vi "DeviceRead.vi"(4 "等待时间（毫秒）":u32, 5 "VISA resource name":refnum<visa-resource-name> caption="VISA资源名称", 6 "写入缓冲区":string, 7 "标准码词":string) -> (0 "错误输出":errorcluster, 1 "x = y?":bool, 2 "数据读取时间":u32, 3 "连接的字符串":string)   [LabVIEW 2020]
uses:
  <vilib>/Instr/_visa.llb/VISA Flush IO Buffer Mask.ctl
  <vilib>/Instr/_visa.llb/VISA Set IO Buffer Mask.ctl
  <vilib>/Instr/_visa.llb/VISA Configure Serial Port (Instr).vi
panel:
  out "读取的数据":string
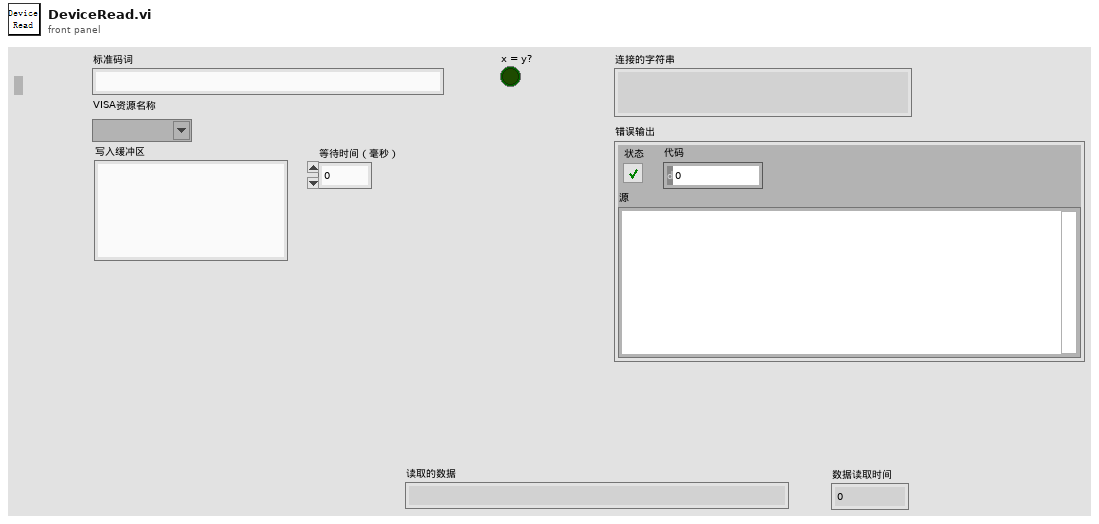
[diagram p1: front panel]
types:
  T1 = typedef "VISA Flush IO Buffer Mask.ctl" = u16
  T2 = typedef "VISA Set IO Buffer Mask.ctl" = u16
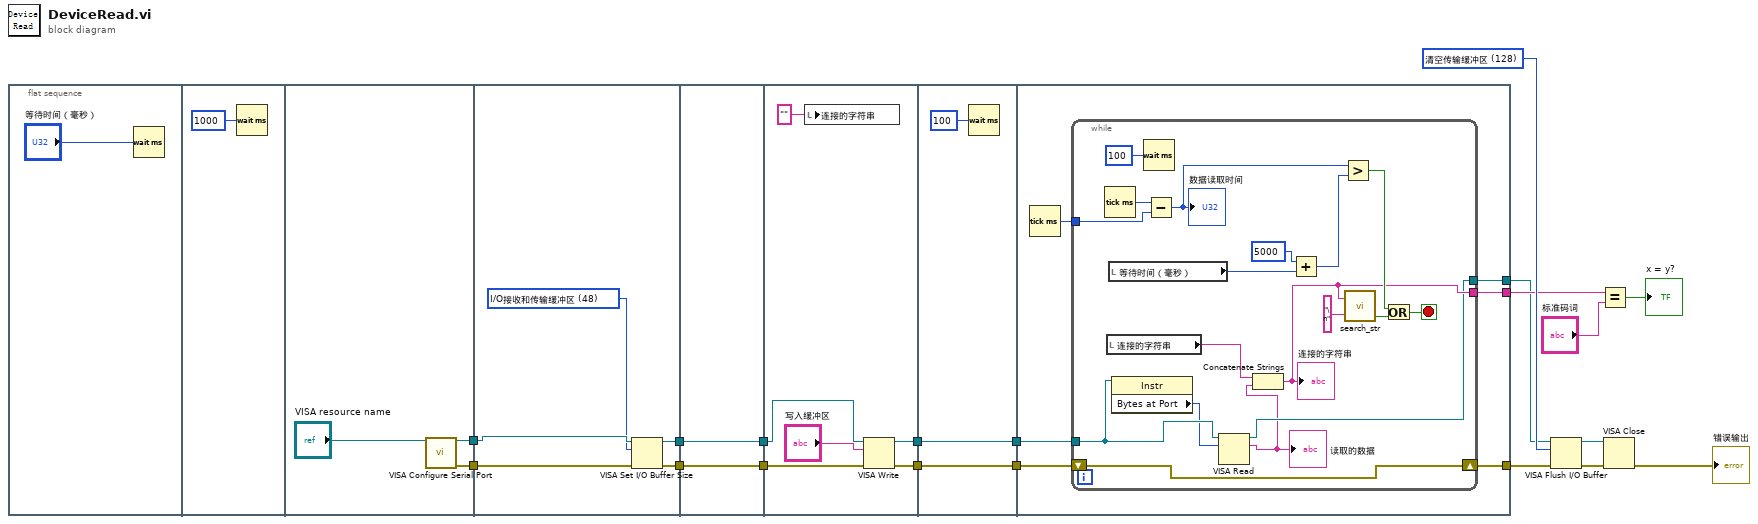
[diagram p0: block diagram]
diagram:
  w13 = T1 128 items=["清空接收缓冲区"=16, "向设备写入传输缓冲区"=32, "清空接收缓冲区（无I/O）"=64, "清空传输缓冲区"=128] ("Mask")
  n1 = flat-sequence {
    tunnel: [w23] -> w2
    tunnel: [w22] -> w1
    tunnel: [w26] -> w4
    tunnel: [w27] -> w3
    tunnel: w2 -> [w29]
    tunnel: w1 -> [w28]
    tunnel: [w31] -> w16
    tunnel: w4 -> [w31]
    tunnel: [w30] -> w15
    tunnel: w3 -> [w30]
    tunnel: [w36] -> w17
    tunnel: w16 -> [w37]
    tunnel: w15 -> [w34]
    tunnel: [w33] -> w11
    tunnel: w17 -> [w39]
    tunnel: w11 -> [w38]
    tunnel: [w39] -> w10
    tunnel: [w38] -> w9
    tunnel: w10 -> [w45]
    tunnel: w9 -> [w44]
    tunnel: [w43] -> w8
    tunnel: [w42] -> w7
    tunnel: [w41] -> w6
    frame #0 {
      n2 = Wait (ms)(milliseconds to wait="等待时间（毫秒）") -> ()  [unwired: 1 out]
    }
    frame #1 {
      n3 = Wait (ms)(milliseconds to wait=u32 1000 ("等待时间（毫秒）")) -> ()  [unwired: 1 out]
    }
    frame #2 {
      n4 = call-poly "VISA Configure Serial Port"("VISA resource name"="VISA resource name") -> ("VISA resource name out"=w22:refnum<visa-resource-name>, "error out"=w23:errorcluster)  [unwired: 13 in]
    }
    frame #3 {
      w25 = T2 48 items=["I/O接收缓冲区"=16, "I/O传输缓冲区"=32, "I/O接收和传输缓冲区"=48] ("Mask")
      n5 = VISA Set I/O Buffer Size(VISA resource name=w28, mask (16)=w25, error in (no error)=w29) -> (VISA resource name out=w26:refnum<visa-resource-name>, error out=w27:errorcluster)  [unwired: 1 in]
    }
    frame #4 {
    }
    frame #5 {
      n6 = local write "连接的字符串"("" ("连接的字符串")) -> ()
      n7 = VISA Write(VISA resource name=w37, write buffer="写入缓冲区", error in (no error)=w34) -> (VISA resource name out=w36:refnum<visa-resource-name>, error out=w33:errorcluster)  [unwired: 1 out]
    }
    frame #6 {
      n8 = Wait (ms)(milliseconds to wait=u32 100 ("等待时间（毫秒）")) -> ()  [unwired: 1 out]
    }
    frame #7 {
      n9 = Tick Count (ms)() -> (millisecond timer value=w46:u32)
      n10 = while {
        tunnel: w46 -> [w62]
        tunnel: [w55] -> w43
        shift-right: [w51] -> w41
        shift-left: w44 -> [w51]
        tunnel: w45 -> [w49]
        tunnel: [w50] -> w42
        stop <- w56 stop-if-true
        n11 = Tick Count (ms)() -> (millisecond timer value=w63:u32)
        n12 = local read "连接的字符串"() -> (w61:string)
        n13 = local read "等待时间（毫秒）"() -> (w53:u32)
        n14 = property class="Instr"(reference=w49) -> ("Bytes at Port"=w48:u32)  [unwired: 1 in, 2 out]
        n15 = Wait (ms)(milliseconds to wait=u32 100 ("等待时间（毫秒）")) -> ()  [unwired: 1 out]
        n16 = Subtract(x=w63, y=w62) -> (x-y=w59:u32)
        "数据读取时间" <- w59
        n17 = VISA Read(VISA resource name=w49, byte count=w48) -> (VISA resource name out=w50:refnum<visa-resource-name>, read buffer=w47:string)  [unwired: 1 in, 2 out]
        "读取的数据" <- w47
        n18 = Concatenate Strings(w61, w47) -> (w55:string)
        "连接的字符串" <- w55
        n19 = Add(x=u32 5000 ("y"), y=w53) -> (x+y=w52:u32)
        n20 = Greater?(x=w59, y=w52) -> (0:w58:bool)
        n21 = call "search_str.vi"("字符串"=w55, "搜索字符串/字符(-)"="\n") -> ("x != y?"=w57:bool)  [unwired: 2 out]
        n22 = Or(x=w58, y=w57) -> (x .or. y?=w56:bool)
      }
    }
  }
  n23 = VISA Flush I/O Buffer(VISA resource name=w7, mask (16)=w13, error in (no error)=w6) -> (VISA resource name out=w12:refnum<visa-resource-name>, error out=w5:errorcluster)
  n24 = Equal?(x=w8, y="标准码词") -> (x = y?=→"x = y?":bool)
  n25 = VISA Close(VISA resource name=w12, error in (no error)=w5) -> (error out=→"错误输出":errorcluster)
